vi "GetSystemBeeperState.vi"(0 "VISA resource name":refnum<visa-resource-name>, 1 "error in (no error)":errorcluster, 3 "Enabled":bool) -> (2 "VISA resource name out":refnum<visa-resource-name>, 4 "error out":errorcluster)   [LabVIEW 2020, in "Active Technologies AWG3000.lvlib"]
uses:
  Active Technologies AWG3000.lvlib
panel:
  out "Beeper State":string
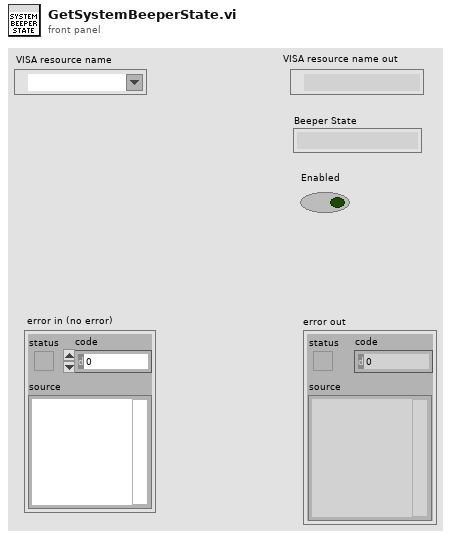
[diagram p1: front panel]
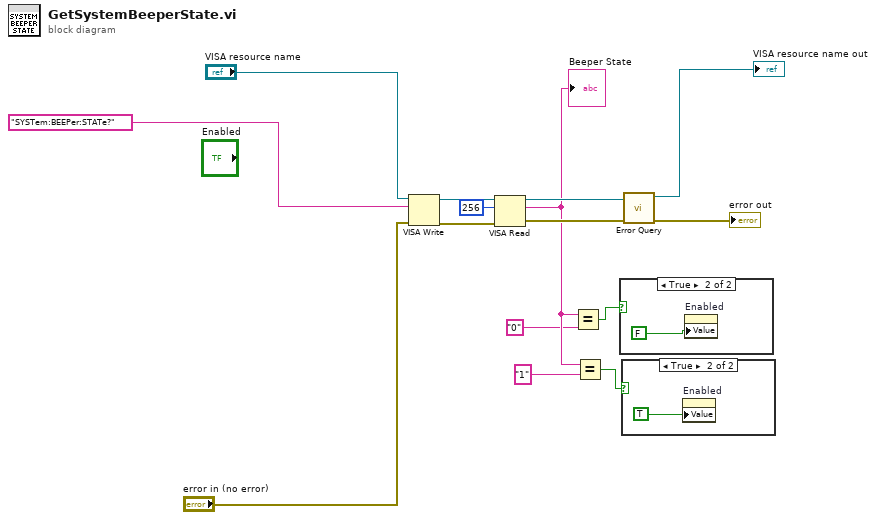
[diagram p0: block diagram]
diagram:
  n1 = VISA Write(VISA resource name="VISA resource name", write buffer="SYSTem:BEEPer:STATe?", error in (no error)="error in (no error)") -> (VISA resource name out=w13:refnum<visa-resource-name>, error out=w12:errorcluster)  [unwired: 1 out]
  n2 = VISA Read(VISA resource name=w13, byte count=u32 256, error in (no error)=w12) -> (VISA resource name out=w10:refnum<visa-resource-name>, read buffer=w3:string, error out=w9:errorcluster)  [unwired: 1 out]
  "Beeper State" <- w3
  n3 = Equal?(x=w3, y="0") -> (x = y?=w5:bool)
  n4 = Equal?(x=w3, y="1") -> (x = y?=w4:bool)
  n5 = case shown="True" w5 {
    frame False {
    }
    frame True {
      n6 = property on="Enabled" class="Bool (strict)"("Value"=FALSE ("CH Polarity positive")) -> ()  [unwired: 2 in, 2 out]
    }
  }
  n7 = case shown="True" w4 {
    frame False {
    }
    frame True {
      n8 = property on="Enabled" class="Bool (strict)"("Value"=TRUE ("CH Polarity positive")) -> ()  [unwired: 2 in, 2 out]
    }
  }
  n9 = call "Error Query.vi"("error in (no error)"=w9, "VISA resource name"=w10) -> ("error out"=→"error out":errorcluster, "VISA resource name out"=→"VISA resource name out":refnum<visa-resource-name>)  [unwired: 6 in, 2 out]
